vi "square joystics.vi"(8 "right joy":dbl, 11 "left joy":dbl) -> (0 "Right Out":dbl, 3 "Left Out":dbl)   [LabVIEW 2016]
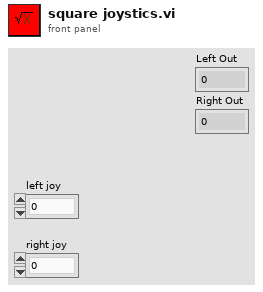
[diagram p1: front panel]
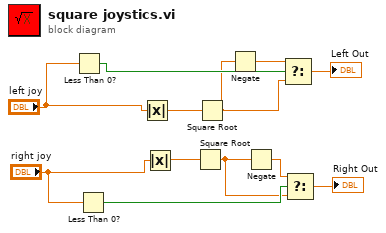
[diagram p0: block diagram]
diagram:
  n1 = Less Than 0?(x="left joy") -> (x < 0?=w7:bool)
  n2 = Less Than 0?(x="right joy") -> (x < 0?=w8:bool)
  n3 = Absolute Value(x="left joy") -> (abs(x)=w12:dbl)
  n4 = Absolute Value(x="right joy") -> (abs(x)=w11:dbl)
  n5 = Square Root(x=w11) -> (sqrt(x)=w4:dbl)
  n6 = Square Root(x=w12) -> (sqrt(x)=w5:dbl)
  n7 = Negate(x=w5) -> (-x=w6:dbl)
  n8 = Negate(x=w4) -> (-x=w3:dbl)
  n9 = Select(t=w6, s=w7, f=w5) -> (s? t:f=→"Left Out":dbl)
  n10 = Select(t=w3, s=w8, f=w4) -> (s? t:f=→"Right Out":dbl)
